vi "Actor Core.vi"(8 "error in":errorcluster, 11 "Function":refnum<class "Function.lvclass">) -> (0 "error out":errorcluster, 3 "Actor out":refnum<class "Actor.lvclass">)   [LabVIEW 2016, in "Function Actor.lvlib" / "Function.lvclass"]
doc: "This is Actor Core.vi, the main message handling loop for Actors. An actor usually just sits in this loop and processes messages as they arrive. Any error returned by the message Do.vi call will stop the loop, with error code 43 as the cannonical signal to stop with no error sent to caller. Descendants may override that in Handle Error.vi."
uses:
  <userlib>/Common Components/Function Actor/Function.lvclass
  C:/Program Files (x86)/National Instruments/LabVIEW 2016/vi.lib/ActorFramework/Actor/Actor.lvclass
  <vilib>/ActorFramework/Actor/Actor.lvclass
  <vilib>/ActorFramework/Actor/Actor.lvclass/Actor.ctl
  <vilib>/ActorFramework/Message Enqueuer/Message Enqueuer.lvclass/Message Enqueuer.ctl
  <userlib>/Common Components/Function Actor/Function.lvclass/Function.ctl
  <userlib>/Common Components/WebSocket Networking/Message 2D String Array/Message 2D String Array.lvclass
  <userlib>/Common Components/Function Messages/Update Connected Clients Msg/Update Connected Clients Msg.lvclass/Update Connected Clients Msg.ctl
  <vilib>/ActorFramework/Message Enqueuer/Init from Existing Queue.vi
  <vilib>/ActorFramework/Message Enqueuer/Enqueue.vi
  <userlib>/Composed Systems/Stream/Mediator/Classes/Message Transport Event/Message Transport Event.lvclass
  C:/Program Files (x86)/National Instruments/LabVIEW 2016/user.lib/Composed Systems/Stream/Mediator/Classes/Message Transport Interface/Message Transport Interface.lvclass
  <userlib>/Common Components/Function Messages/Update Connected Clients Msg/Update Connected Clients Msg.lvclass
  C:/Program Files (x86)/National Instruments/LabVIEW 2016/vi.lib/ActorFramework/Message/Message.lvclass
  <vilib>/ActorFramework/Stop Msg/Stop Msg.lvclass
  <vilib>/ActorFramework/Message Priority Queue/Priority Enqueue.vi
  <vilib>/ActorFramework/Message Enqueuer/Message Enqueuer.lvclass
  <userlib>/Common Components/WebSocket Networking/WS Message Broker Interface Ref/WS Message Broker Interface Ref.lvclass
panel:
  out "Connected Clients":i32(listbox)
  out "Cmd List":i32(listbox)
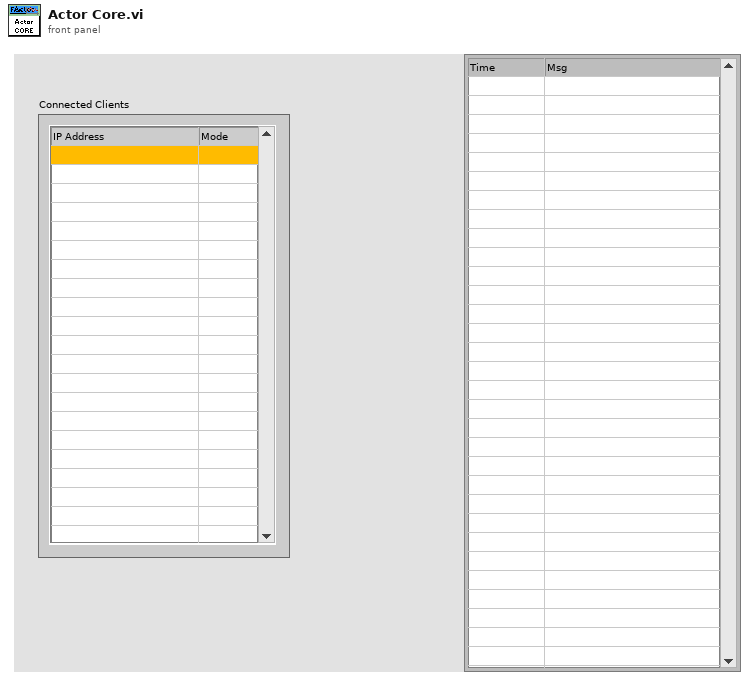
[diagram p1: front panel]
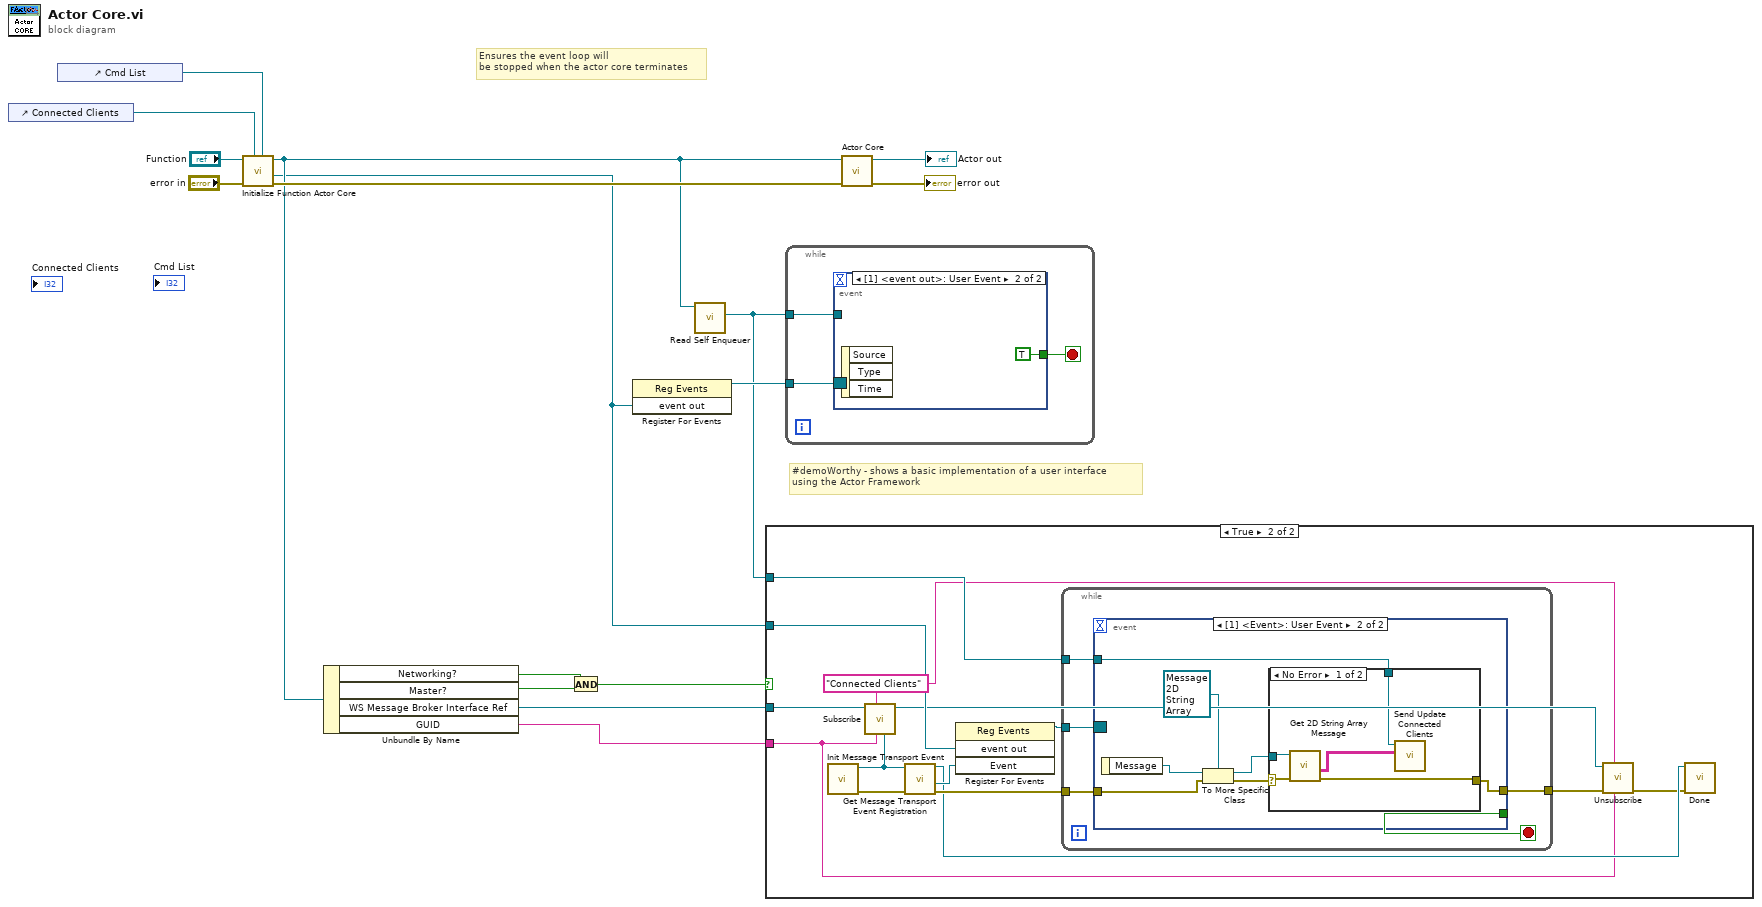
[diagram p0: block diagram]
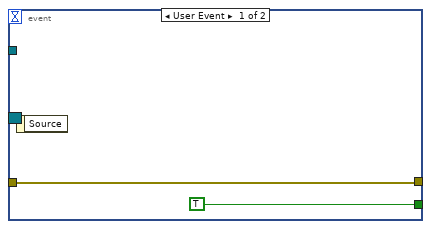
[diagram p3: hidden frame]
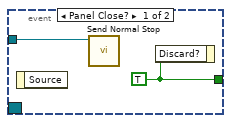
[diagram p5: hidden frame]
diagram:
  # "#demoWorthy - shows a basic implementation of a user interface\nusing the Actor Framework"
  # "Ensures the event loop will \nbe stopped when the actor core terminates"
  n1 = control-ref of="Connected Clients"() -> (w9:refnum<vi>)
  n2 = control-ref of="Cmd List"() -> (w10:refnum<vi>)
  n3 = call <userlib>:"Initialize Function Actor Core.vi"("Cmd List"=w10, "Connected Clients"=w9, "error in (no error)"="error in", "Function in"="Function") -> ("error out"=w11:errorcluster, "event out"=w3:refnum<user-event>, "Function out"=w8:refnum<class "Function.lvclass">)  [unwired: 4 in, 1 out]
  n4 = Unbundle By Name(w8) -> ("Networking?"=w7:bool, "Master?"=w6:bool, "WS Message Broker Interface Ref"=w4:refnum<class "WS Message Broker Interface Ref.lvclass">, "GUID"=w1:string)
  n5 = And(x=w7, y=w6) -> (x .and. y?=w5:bool)
  n6 = register-events(w3) -> (reference out=w12:refnum<event-registration>)  [unwired: 2 in, 1 out]
  n7 = call <vilib>:"Read Self Enqueuer.vi"("Actor"=w8) -> ("Self Enqueuer"=w2:refnum<class "Message Enqueuer.lvclass">)  [unwired: 10 in]
  n8 = case shown="True" w5 {
    tunnel: w4 -> [_ w28]
    tunnel: w3 -> [_ w27]
    tunnel: w2 -> [_ w21]
    tunnel: w1 -> [_ w17]
    frame False {
    }
    frame True {
      w18 = "Connected Clients" ("Topic Name")
      n9 = call <userlib>:"Init Message Transport Event.vi"() -> ("error out"=w29:errorcluster, "Message Transport Event out"=w30:refnum<class "Message Transport Event.lvclass">)  [unwired: 10 in]
      n10 = call-dynamic "Subscribe.vi"("Message Transport Interface"=w30, "Subscriber Name"=w17, "Topic Name"=w18, "Message Broker Interface TAP in"=w28) -> ("Message Broker Interface TAP out"=w19:refnum<class "WS Message Broker Interface Ref.lvclass">)  [unwired: 5 in, 2 out]
      n11 = call <userlib>:"Get Message Transport Event Registration.vi"("error in (no error)"=w29, "Message Transport Event in"=w30) -> ("error out"=w24:errorcluster, "Event"=w26:refnum<user-event>, "Message Transport Event out"=w22:refnum<class "Message Transport Event.lvclass">)  [unwired: 6 in, 1 out]
      n12 = register-events(w27, w26) -> (reference out=w25:refnum<event-registration>)  [unwired: 2 in, 1 out]
      n13 = while {
        tunnel: w25 -> [w35]
        tunnel: w24 -> [w33]
        tunnel: [w32] -> w23
        tunnel: w21 -> [w31]
        stop <- w34 stop-if-true
        n14 = event shown="[1] <Event>: User Event" {
          selector: w35 -> [_ _]
          dyn-events: _ -> [_ _]
          timeout: _ -> [_ _]
          tunnel: [TRUE _] -> w34
          tunnel: w33 -> [w36 w40]
          tunnel: [w36 w39] -> w32
          tunnel: w31 -> [_ w38]
          event User Event {
            n15 = event-data() -> ()  [unwired: 1 in, 1 out]
          }
          event User Event {
            n16 = event-data() -> ("Message"=w41:refnum<class "Message Interface.lvclass">)  [unwired: 1 in]
            n17 = To More Specific Class(target class=refnum<class "Message 2D String Array.lvclass"> refnum ("Stream Mediator.lvlib:Message 2D String Array.lvclass"), reference=w41, error in=w40) -> (specific class reference=w43:refnum<class "Message 2D String Array.lvclass">, error out=w44:errorcluster)
            n18 = case shown="No Error" w44 {
              selector: w44 -> [w48 w50]
              tunnel: [w47 w50] -> w39
              tunnel: w43 -> [w49 _]
              tunnel: w38 -> [w46 _]
              frame No Error {
                n19 = call <userlib>:"Get 2D String Array Message.vi"("error in (no error)"=w48, "Message Double in"=w49) -> ("error out"=w47:errorcluster, "Value"=w45:string[][])  [unwired: 6 in, 2 out]
                n20 = call <userlib>:"Send Update Connected Clients.vi"("2D Array of String"=w45, "Message Enqueuer"=w46) -> ()  [unwired: 8 in, 2 out]
              }
              frame Error {
              }
            }
          }
        }
      }
      n21 = call-dynamic "Unsubscribe.vi"("Subscriber Name"=w17, "Topic Name"=w18, "error in (no error)"=w23, "Message Broker Interface TAP in"=w19) -> ("error out"=w20:errorcluster)  [unwired: 6 in, 1 out]
      n22 = call-dynamic "Done.vi"("error in (no error)"=w20, "Message Transport Event in"=w22) -> ()  [unwired: 8 in, 2 out]
    }
  }
  n23 = while {
    tunnel: w2 -> [w53]
    tunnel: w12 -> [w51]
    stop <- w52 stop-if-true
    n24 = event shown="[1] <event out>: User Event" {
      selector: w51 -> [_ _]
      dyn-events: _ -> [_ _]
      timeout: _ -> [_ _]
      tunnel: w53 -> [w54 _]
      tunnel: [w55 TRUE ("Discard?")] -> w52
      event Panel Close? {
        w55 = TRUE ("Discard?")
        n25 = event-data() -> ()  [unwired: 1 in, 1 out]
        n26 = call <vilib>:"Send Normal Stop.vi"("Message Enqueuer"=w54) -> ()  [unwired: 10 in, 1 out]
        n27 = event-data("Discard?"=w55) -> ()  [unwired: 1 in, 1 out]
      }
      event User Event {
        n28 = event-data() -> ()  [unwired: 1 in, 3 out]
      }
    }
  }
  n29 = call-parent "Actor Core.vi"("error in"=w11, "Actor in"=w8) -> ("error out"=→"error out":errorcluster, "Actor out"=→"Actor out":refnum<class "Actor.lvclass">)  [unwired: 8 in]
